vi "image to RGB array.vi"(11 "Image Pixels (U32)":u32[][](array[numeric])) -> (3 "Image Pixels (U8)":u8[][][](array[numeric]))   [LabVIEW 2017]
doc: "Separates a 320x240 array of U32 pixels into their RGB components. The result is a 3x320x240 array of U8 pixels, with a page for red, a page for green, and a page for blue."
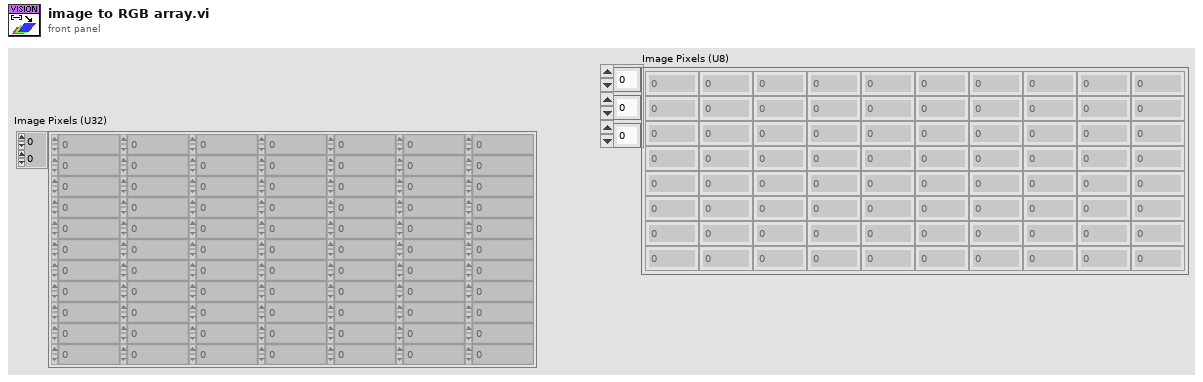
[diagram p1: front panel]
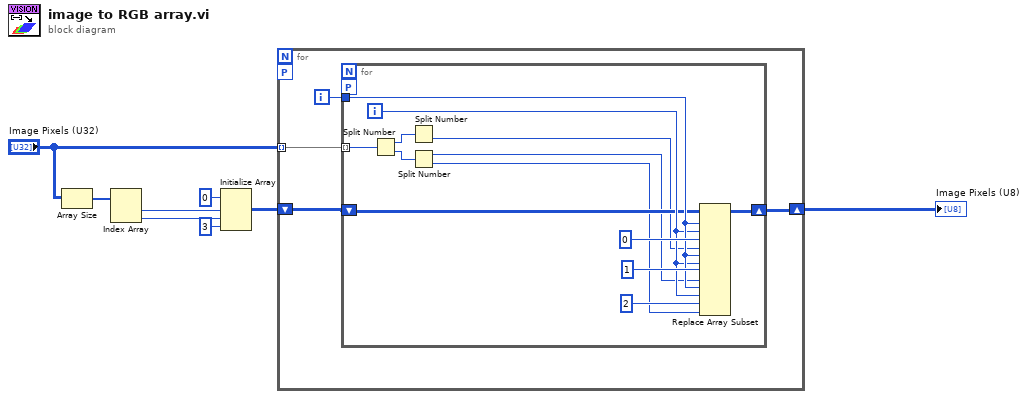
[diagram p0: block diagram]
diagram:
  n1 = Array Size(array="Image Pixels (U32)") -> (size(s)=w3:i32[])
  n2 = Index Array(array=w3) -> (element #1=w2:i32, element #2=w1:i32)  [unwired: 2 in]
  n3 = Initialize Array(u8 0 ("element"), w2, w1, 3 ("dimension size")) -> (w6:u8[][][])
  n4 = for {
    tunnel: "Image Pixels (U32)" -> [w12] mode=indexing
    shift-right: [w10] -> w5
    shift-left: w6 -> [w11]
    workers-P: _ -> [_]
    i -> [w9]
    n5 = for {
      tunnel: w12 -> [w18] mode=indexing
      shift-right: [w24] -> w10
      shift-left: w11 -> [w19]
      tunnel: w9 -> [w22]
      workers-P: _ -> [_]
      i -> [w21]
      n6 = Split Number(x=w18) -> (hi(x)=w17:u16, lo(x)=w16:u16)
      n7 = Split Number(x=w17) -> (lo(x)=w15:u8)  [unwired: 1 out]
      n8 = Split Number(x=w16) -> (hi(x)=w14:u8, lo(x)=w13:u8)
      n9 = Replace Array Subset(array=w19, new element #1=w15, index (dim 0) #1=w22, index (dim 1) #1=w21, index (dim 2) #1=0 ("disabled index (col)"), new element #2=w14, index (dim 0) #2=w22, index (dim 1) #2=w21, index (dim 2) #2=1 ("disabled index (col)"), new element #3=w13, index (dim 0) #3=w22, index (dim 1) #3=w21, index (dim 2) #3=2 ("disabled index (col)")) -> (w24:u8[][][])
    }
  }
  "Image Pixels (U8)" <- w5
